vi "fgv_hw-info.vi"(7 "cmd":enum16{"write", "read"}(ring), 11 "HW info":T1={"UGV"=enum."Scout", "Lidar 1"=enum."none", "Lidar 2"=enum."none", "GPS"=enum."none", "Camera 1"=enum."none", "Joystick"=enum."none", "sound"=enum."none", "IMU"=enum."none", "Led"=enum."none", "Camera 2"=enum."none", "Camera 3"=enum."none", "Camera 4"=enum."none"}) -> (3 "HW info out":T1={"UGV"=enum."Scout", "Lidar 1"=enum."none", "Lidar 2"=enum."none", "GPS"=enum."none", "Camera 1"=enum."none", "Joystick"=enum."none", "sound"=enum."none", "IMU"=enum."none", "Led"=enum."none", "Camera 2"=enum."none", "Camera 3"=enum."none", "Camera 4"=enum."none"})   [LabVIEW 2021]
uses:
  Ctrl/system_hw.ctl
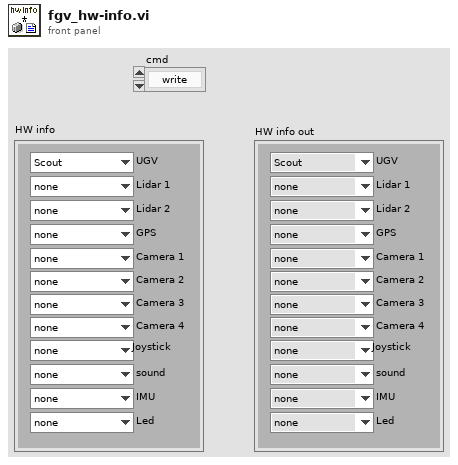
[diagram p1: front panel]
types:
  T1 = typedef "system_hw.ctl" = cluster{"UGV":enum16{"none", "Scout", "RLCar", "ASV", "Bunker"}, "Lidar 1":enum16{"none", "VLP16", "TIM571", "RPLidar A2", "RPLidar A3", "Ouster"}, "Lidar 2":enum16{"none", "VLP16", "TIM571", "RPLidar A2", "RPLidar A3"}, "GPS":enum16{"none", "NMEA 232", "Custom", "tbd"}, "Camera 1":enum16{"none", "C920", "C922", "GT1290C", "MS LifeCam"}, "Joystick":enum16{"none", "joystick"}, "sound":enum16{"none", "speaker"}, "IMU":enum16{"none", "MW-AHRSv1", "VN-100", "MTi-630", "Ellipse-D", "WT901CTTL"}, "Led":enum16{"none", "LedMatrix 8x32"}, "Camera 2":enum16{"none", "C920", "C922", "GT1290C", "MS LifeCam"}, "Camera 3":enum16{"none", "C920", "C922", "GT1290C", "MS LifeCam"}, "Camera 4":enum16{"none", "C920", "C922", "GT1290C", "MS LifeCam"}}
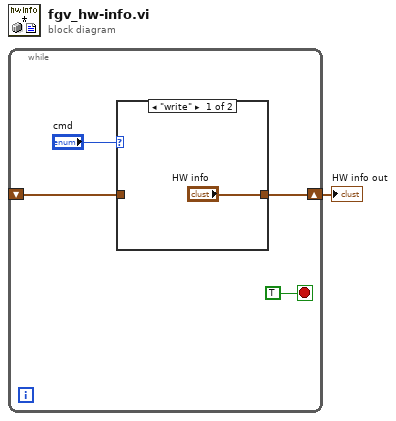
[diagram p0: block diagram]
diagram:
  n1 = while {
    shift-right: [w3] -> w1
    shift-left: _ -> [w2]
    stop <- TRUE stop-if-true
    n2 = case shown="\"write\"" "cmd" {
      tunnel: ["HW info" w7] -> w3
      tunnel: w2 -> [_ w7]
      frame "write" {
      }
      frame "read", Default {
      }
    }
  }
  "HW info out" <- w1
